vi "N次方根（牛顿迭代法）.vi"() -> ()   [LabVIEW 2012]
doc: "功能：\n\n利用牛顿迭代法求一个数的n次方根\n\n\ncsxcs_366创建"
uses:
  <vilib>/express/express arith-compare/Formula/XNode/ExpressFormulaBlockNode.xnode
panel:
  in  "m":dbl
  out "n-th root(x)":dbl
  in  "x":dbl
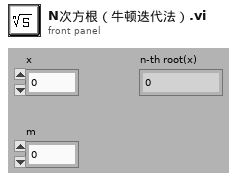
[diagram p1: front panel]
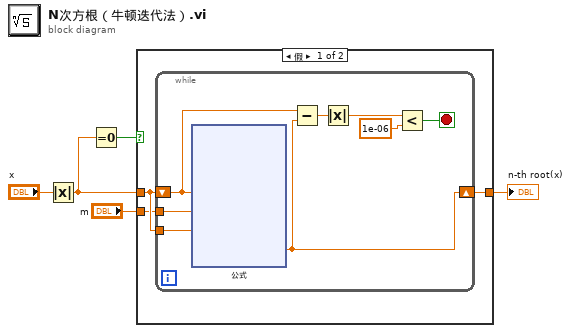
[diagram p0: block diagram]
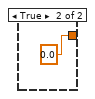
[diagram p2: hidden frame]
diagram:
  n1 = Absolute Value(x="x") -> (abs(x)=w1:dbl)
  n2 = Equal To 0?(x=w1) -> (x = 0?=w4:bool)
  n3 = case shown="假" w4 {
    tunnel: w1 -> [w7 _]
    tunnel: [w8 0.0 ("x")] -> w3
    tunnel: "m" -> [w6 _]
    frame False {
      n4 = while {
        shift-right: [w10] -> w8
        shift-left: w7 -> [w9]
        tunnel: w7 -> [w12]
        tunnel: w6 -> [w13]
        stop <- w14 stop-if-true
        n5 = xnode "公式"("Xn"=w9, "m"=w13, "a"=w12) -> ("结果"=w10:dbl)  [unwired: 1 in, 1 out]
        n6 = Subtract(x=w9, y=w10) -> (x-y=w11:dbl)
        n7 = Absolute Value(x=w11) -> (abs(x)=w16:dbl)
        n8 = Less?(x=w16, y=1e-06) -> (x < y?=w14:bool)
      }
    }
    frame True {
    }
  }
  "n-th root(x)" <- w3
